vi "LIN Get Key.vi"(1 "x":u16 format="%.0x") -> (0 "KEY":u8[](array[numeric]) format="%.0x")   [LabVIEW 2018]
panel:
  out "lo(x)":u8 format="%.0x"
  out "hi(x)":u8 format="%.0x"
  out "y":u16 format="%.0x"
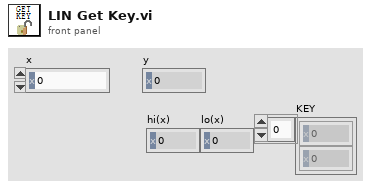
[diagram p1: front panel]
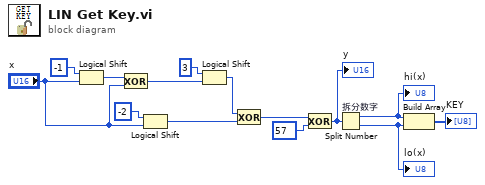
[diagram p0: block diagram]
diagram:
  n1 = Logical Shift ("逻辑移位")(y=i16 -1, x="x") -> (x << y=w13:u16)
  n2 = Exclusive Or ("异或")(1:"x", 2:w13) -> (0:w12:u16)
  n3 = Logical Shift(y=i16 -2, x="x") -> (x << y=w8:u16)
  n4 = Logical Shift(y=i16 3, x=w12) -> (x << y=w7:u16)
  n5 = Exclusive Or(1:w8, 2:w7) -> (0:w6:u16)
  n6 = Exclusive Or(1:u16 57 ("y"), 2:w6) -> (0:w4:u16)
  "y" <- w4
  n7 = Split Number "拆分数字"(x=w4) -> (hi(x)=w3:u8, lo(x)=w2:u8)
  "hi(x)" <- w3
  "lo(x)" <- w2
  n8 = Build Array(w3, w2) -> (→"KEY":u8[])
